vi "Temperature Monitor.vi"() -> ()   [LabVIEW 2022 SP3]
panel:
  in  "Thermometer":dbl(slide) scale=0.0..100.0
  out "Temperature History":dbl(graph)
  in  "stop":bool
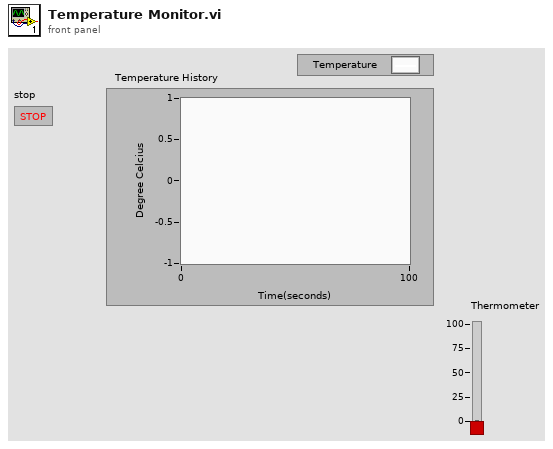
[diagram p1: front panel]
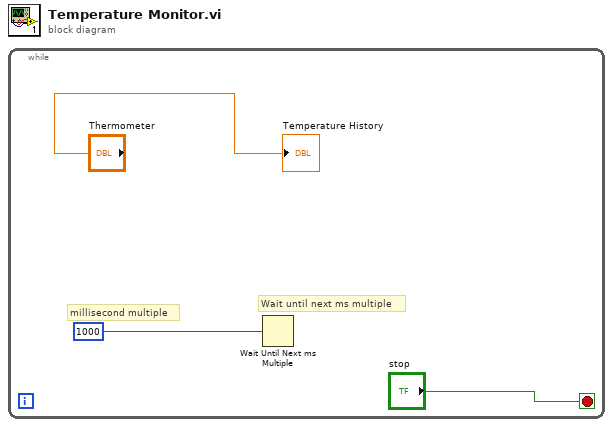
[diagram p0: block diagram]
diagram:
  n1 = while {
    stop <- "stop" stop-if-true
    # "Wait until next ms multiple"
    # "millisecond multiple"
    n2 = Wait Until Next ms Multiple(millisecond multiple=u32 1000) -> ()  [unwired: 1 out]
    "Temperature History" <- "Thermometer"
  }
